vi "locate channel in module.vi"(8 "error in":errorcluster, 9 "channel name":string, 10 "instance id":string, 11 "Modules Configurations":refnum<class "TBM module configuration.lvclass">[](array[class])) -> (0 "error out":errorcluster, 3 "channel":refnum<class "TBM channel.lvclass">)   [LabVIEW 2013, in "PL Framework Configuration Tool.lvlib" / "Engine Mappings.lvclass"]
uses:
  Engine Mappings.lvclass
  <vilib>/NI/Tag Bus Module Framework/channel/TBM channel.lvclass
  <vilib>/NI/Tag Bus Module Framework/module configuration/TBM module configuration.lvclass
  <vilib>/NI/CEF/CEF_TreeControl/serializable configuration/NISE_CEF_serializable configuration.lvclass/NISE_CEF_serializable configuration.ctl
  <vilib>/NI/CEF/CEF_TreeControl/serializable configuration/NISE_CEF_serializable configuration.lvclass
  <vilib>/NI/Tag Bus/tag/tag descriptor.lvclass/tag descriptor.ctl
  <vilib>/NI/CEF/CEF_TreeControl/serializable configuration/Read UID.vi
  <vilib>/NI/Tag Bus/tag/read tag name.vi
  <vilib>/NI/Tag Bus Module Framework/root configuration/TBM configuration.lvclass
  <vilib>/NI/Tag Bus/tag/tag descriptor.lvclass
  <vilib>/NI/CEF/CEF_TreeControl/NISE_CEF_TreeControl.lvlib
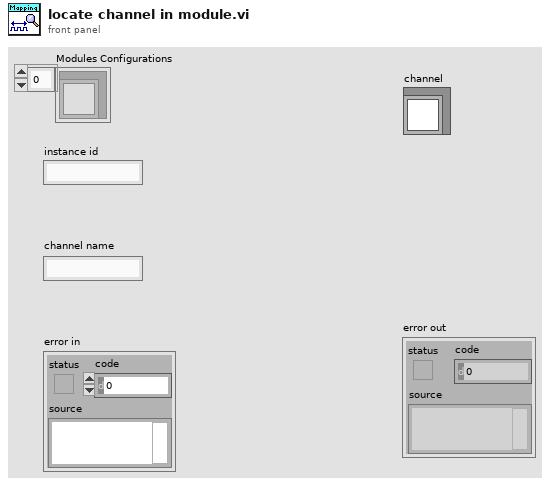
[diagram p1: front panel]
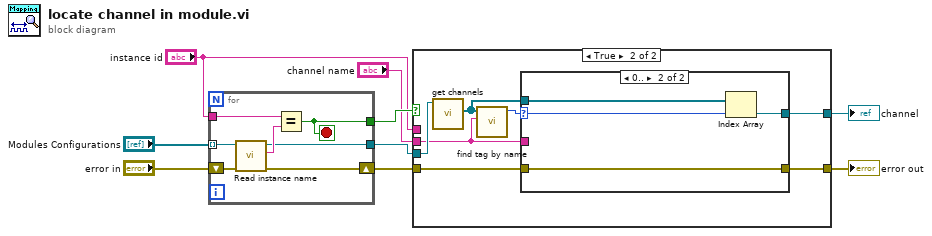
[diagram p0: block diagram]
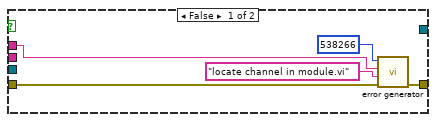
[diagram p2: hidden frame]
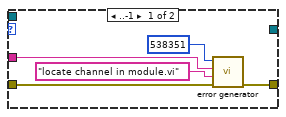
[diagram p3: hidden frame]
diagram:
  n1 = for {
    tunnel: "Modules Configurations" -> [w16] mode=indexing
    tunnel: "instance id" -> [w13]
    tunnel: [w12] -> w6
    shift-right: [w11] -> w8
    shift-left: "error in" -> [w15]
    tunnel: [w10] -> w9
    stop <- w10 stop-if-true
    n2 = call <vilib>:"Read instance name.vi"("error in"=w15, "configuration in"=w16) -> ("error out"=w11:errorcluster, "instance id"=w14:string, "configuration out"=w12:refnum<class "TBM module configuration.lvclass">)  [unwired: 7 in]
    n3 = Equal?(x=w13, y=w14) -> (x = y?=w10:bool)
  }
  n4 = case shown="True" w9 {
    tunnel: w8 -> [w21 w24]
    tunnel: "instance id" -> [w20 _]
    tunnel: [w17 w23] -> w7
    tunnel: w6 -> [_ w28]
    tunnel: "channel name" -> [_ w22]
    tunnel: [_ w25] -> w3
    frame False {
      n5 = call <vilib>:"error generator.vi"("error in"=w21, "source"="locate channel in module.vi", "append error message"=w20, "error code (0)"=538266) -> ("error out"=w17:errorcluster)  [unwired: 5 in]
    }
    frame True {
      n6 = call-dynamic "get channels.vi"("module configuration in"=w28) -> ("channels"=w26:refnum<class "TBM channel.lvclass">[])  [unwired: 9 in, 1 out]
      n7 = call <vilib>:"find tag by name.vi"("name"=w22, "tags in"=w26) -> ("index"=w27:i32)  [unwired: 9 in]
      n8 = case shown="0.." w27 {
        selector: w27 -> [_ w36]
        tunnel: w26 -> [_ w37]
        tunnel: [_ w35] -> w25
        tunnel: w24 -> [w30 w34]
        tunnel: [w31 w34] -> w23
        tunnel: w22 -> [w29 _]
        frame ..-1 {
          n9 = call <vilib>:"error generator.vi"("error in"=w30, "source"="locate channel in module.vi", "append error message"=w29, "error code (0)"=538351) -> ("error out"=w31:errorcluster)  [unwired: 5 in]
        }
        frame 0.. {
          n10 = Index Array(array=w37, index=w36) -> (element=w35:refnum<class "TBM channel.lvclass">)
        }
      }
    }
  }
  "error out" <- w7
  "channel" <- w3
